vi "Update State.vi"(8 "error in (no error)":errorcluster, 10 "Open?":bool, 11 "Valve in":refnum<class "Valve.lvclass">) -> (0 "error out":errorcluster, 3 "Valve out":refnum<class "Valve.lvclass">)   [LabVIEW 2021, in "Valve.lvlib" / "Valve.lvclass"]
uses:
  Valve.lvclass
  Valve.lvclass/Valve.ctl
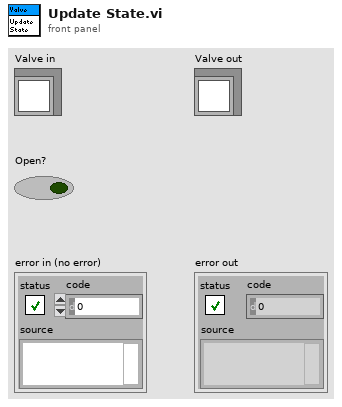
[diagram p1: front panel]
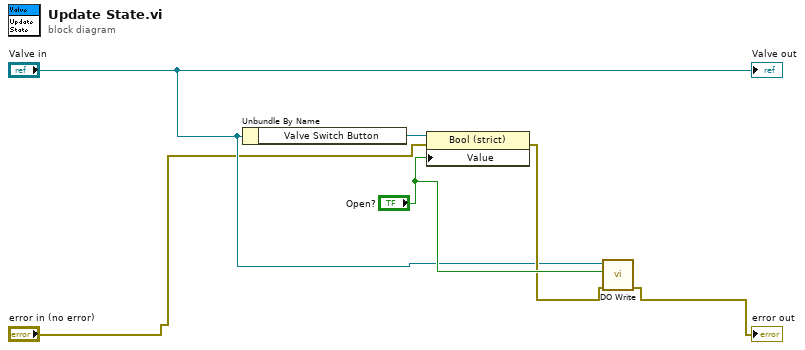
[diagram p0: block diagram]
diagram:
  n1 = Unbundle By Name("Valve in") -> ("Valve Switch Button"=w6:refnum<vi>)
  n2 = property class="Bool (strict)"(reference=w6, error in="error in (no error)", "Value"="Open?") -> (error out=w4:errorcluster)  [unwired: 1 out]
  n3 = call "DO Write.vi"("error in (no error)"=w4, "Digital Output"="Open?", "Valve in"="Valve in") -> ("error out"=→"error out":errorcluster)  [unwired: 8 in]
  "Valve out" <- "Valve in"
